vi "Post-Dig.vi"(6 "Search Path":path[](array[path]), 8 "Error In":errorcluster, 10 "Grave In":refnum<vi>, 11 "VI In":refnum<vi>) -> (0 "Error Out":errorcluster, 2 "Grave Out":refnum<vi>, 3 "VI Out":refnum<vi>)   [LabVIEW 2018, in "Toolkit.lvlib"]
uses:
  Toolkit.lvlib
  Typedefs/Hooks.ctl
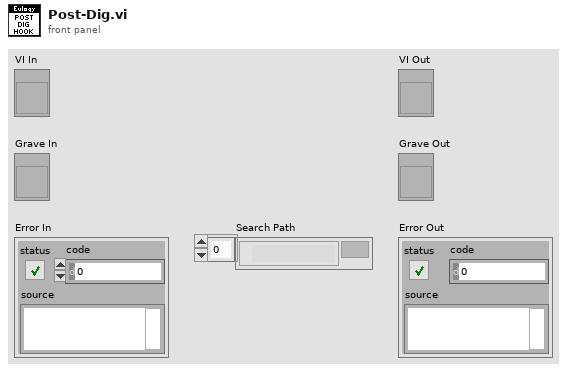
[diagram p1: front panel]
types:
  T1 = typedef "Toolkit.lvlib/Hooks.ctl" = enum16{"Pre-Bury", "Post-Bury", "Pre-Dig", "Post-Dig", "Pre-Reanimate", "Post-Reanimate", "Pre-Smite", "Post-Smite"}
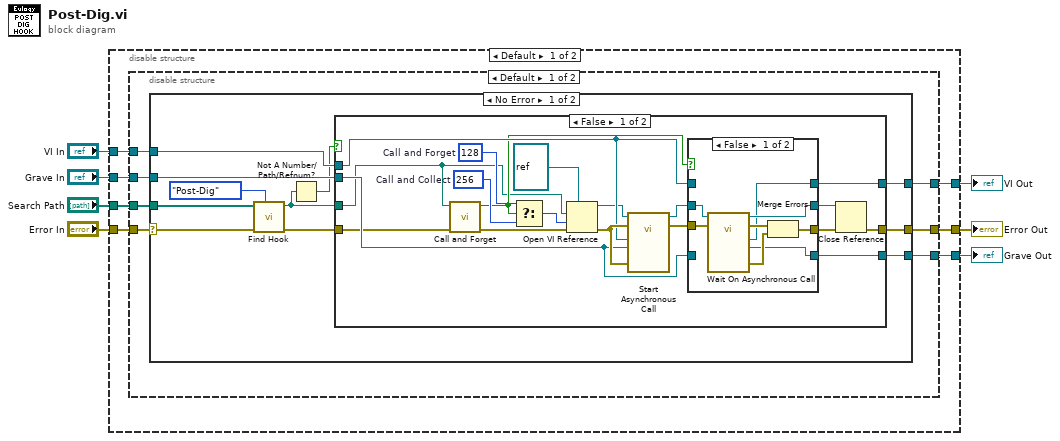
[diagram p0: block diagram]
diagram:
  n1 = disable-structure "Conditional Disable Structure" shown="Default" {
    disable-tunnel: [w14 w74] -> w7
    disable-tunnel: "VI In" -> [w13 w75]
    disable-tunnel: "Error In" -> [w12 w74]
    disable-tunnel: [w11 w75] -> w4
    disable-tunnel: "Search Path" -> [w10 _]
    disable-tunnel: "Grave In" -> [w9 w73]
    disable-tunnel: [w8 w73] -> w1
    frame condition #0 (active) {
      n2 = disable-structure "Conditional Disable Structure" shown="Default" {
        disable-tunnel: [w21 w70] -> w14
        disable-tunnel: w13 -> [w20 w72]
        disable-tunnel: w12 -> [w19 w70]
        disable-tunnel: [w18 w72] -> w11
        disable-tunnel: w10 -> [w17 _]
        disable-tunnel: w9 -> [w16 w71]
        disable-tunnel: [w15 w71] -> w8
        frame condition #0 (active) {
          n3 = case shown="No Error" w19 {
            selector: w19 -> [w30 w69]
            tunnel: [w31 w69] -> w21
            tunnel: w20 -> [w27 w68]
            tunnel: [w29 w67] -> w15
            tunnel: [w28 w68] -> w18
            tunnel: w17 -> [w23 _]
            tunnel: w16 -> [w26 w67]
            frame No Error {
              n4 = call "Find Hook.vi"("Hook"=Hooks."Post-Dig", "Error In"=w30, "Search Path"=w23) -> ("Error Out"=w32:errorcluster, "Hook"=w25:path)  [unwired: 7 in]
              n5 = Not A Number/Path/Refnum?(number/path/refnum=w25) -> (NaN/Path/Refnum?=w24:bool)
              n6 = case shown="False" w24 {
                tunnel: w25 -> [w35 _]
                tunnel: w32 -> [w38 w65]
                tunnel: [w51 w65] -> w31
                tunnel: [w45 w64] -> w29
                tunnel: [w44 w66] -> w28
                tunnel: w27 -> [w43 w66]
                tunnel: w26 -> [w39 w64]
                frame False {
                  w41 = 256  # Call and Collect
                  w42 = 128  # Call and Forget
                  n7 = call "Call and Forget.vi"("Error In"=w38, "Hook"=w35) -> ("Error Out"=w37:errorcluster, "Call and Forget"=w36:bool)  [unwired: 8 in]
                  n8 = Select(t=w42, s=w36, f=w41) -> (s? t:f=w40:i32)
                  n9 = Open VI Reference(type specifier VI Refnum (for type only)=refnum<vi> refnum, vi path=w35, options=w40, error in (no error)=w37) -> (vi reference=w33:refnum<vi>, error out=w50:errorcluster)  [unwired: 2 in]
                  n10 = call-by-ref "Start Asynchronous Call"(reference=w33, error in=w50, "Error In"=w50, "Grave In"=w39, "VI In"=w43) -> (reference out=w49:refnum<vi>, error out=w47:errorcluster)  [unwired: 6 in, 3 out]
                  n11 = case shown="False" w36 {
                    tunnel: w49 -> [w59 w63]
                    tunnel: [w58 w63] -> w48
                    tunnel: w47 -> [w57 w62]
                    tunnel: [w55 w62] -> w46
                    tunnel: [w53 w60] -> w45
                    tunnel: [w52 w61] -> w44
                    tunnel: w43 -> [_ w61]
                    tunnel: w39 -> [_ w60]
                    frame False {
                      n12 = call-by-ref "Wait On Asynchronous Call"(reference=w59, error in=w57) -> (reference out=w58:refnum<vi>, error out=w56:errorcluster, "Error Out"=w54:errorcluster, "Grave Out"=w53:refnum<vi>, "VI Out"=w52:refnum<vi>)  [unwired: 9 in]
                      n13 = Merge Errors(w56, w54) -> (w55:errorcluster)
                    }
                    frame True {
                    }
                  }
                  n14 = Close Reference(reference=w48, error in (no error)=w46) -> (error out=w51:errorcluster)
                }
                frame True {
                }
              }
            }
            frame Error {
            }
          }
        }
        frame condition #1 {
        }
      }
    }
    frame condition #1 {
    }
  }
  "Error Out" <- w7
  "VI Out" <- w4
  "Grave Out" <- w1
